vi "FindAndTrackFaces.vi"(7 "Check face":bool, 8 "error in (no error)":errorcluster, 10 "Image in":T1, 11 "Object Tracking Session In":T2) -> (0 "error out":errorcluster, 1 "Face Images":T1[](array[typedef]), 2 "Image out":T1(plugin-control), 3 "Object Tracking Session Out":T2)   [LabVIEW 2019]
uses:
  <vilib>/vision/Image Controls.llb/IMAQ Image.ctl
  <vilib>/vision/Tracking.llb/IMAQ Object Tracking Session.ctl
panel:
  out "size(s)":i32
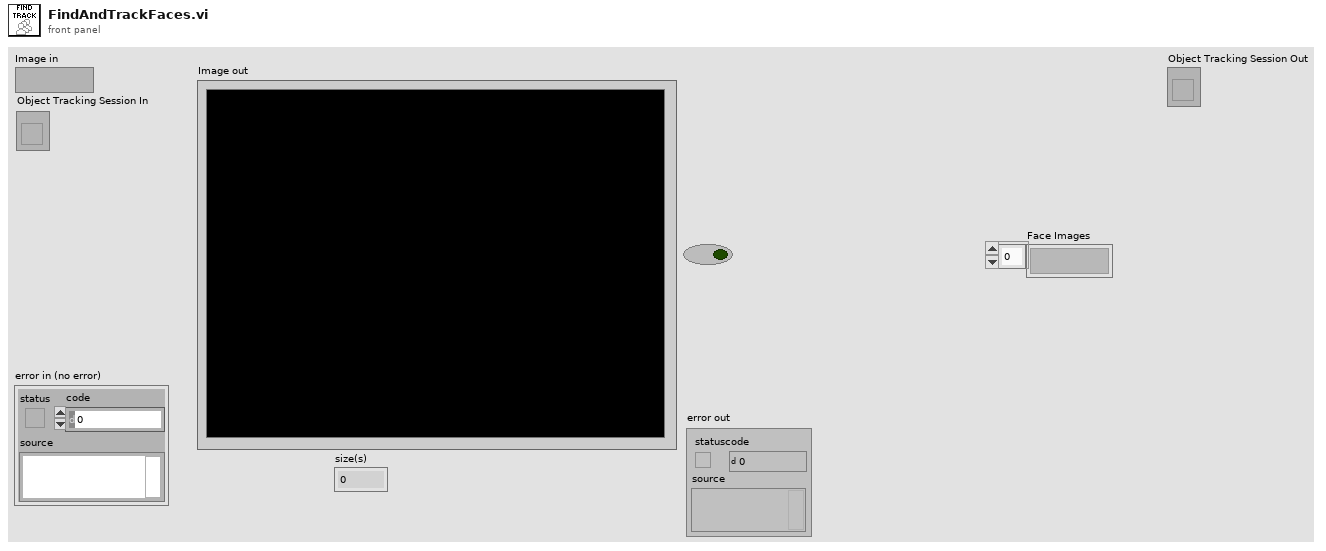
[diagram p1: front panel]
types:
  T1 = typedef "IMAQ Image.ctl" = refnum<image>
  T2 = typedef "IMAQ Object Tracking Session.ctl" = refnum<k20>
  T3 = typedef "IMAQ Rectangle" = cluster{"Left":i32, "Top":i32, "Right":i32, "Bottom":i32, "Rotation":dbl}
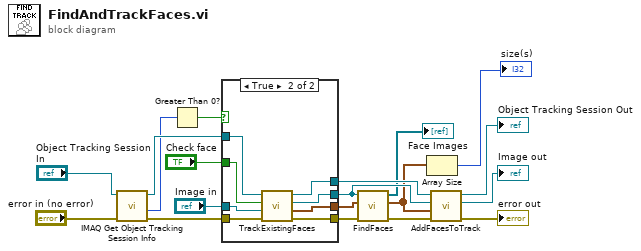
[diagram p0: block diagram]
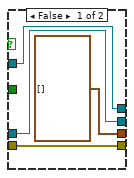
[diagram p2: hidden frame]
diagram:
  n1 = call "IMAQ Get Object Tracking Session Info"("error in (no error)"="error in (no error)", "Object Tracking Session In"="Object Tracking Session In") -> ("error out"=w10:errorcluster, "Number of Objects"=w11:i32, "Object Tracking Session Out"=w13:T2)  [unwired: 6 in, 1 out]
  n2 = Greater Than 0?(x=w11) -> (x > 0?=w12:bool)
  n3 = case shown="True" w12 {
    tunnel: "Image in" -> [w22 w31]
    tunnel: w13 -> [w23 w30]
    tunnel: w10 -> [w21 w29]
    tunnel: [w21 w28] -> w18
    tunnel: [w22 w27] -> w9
    tunnel: [w23 w26] -> w16
    tunnel: [T3[] [] w25] -> w8
    tunnel: "Check face" -> [_ w24]
    frame False {
    }
    frame True {
      n4 = call "TrackExistingFaces.vi"("error in (no error)"=w29, "Image in"=w31, "Check face"=w24, "Refnum in"=w30) -> ("error out"=w28:errorcluster, "Array"=w25:T3[], "Image (duplicate)"=w27:T1, "Refnum out"=w26:T2)  [unwired: 4 in]
    }
  }
  n5 = call "FindFaces.vi"("error in"=w18, "Faces In"=w8, "Image In"=w9) -> ("error out"=w15:errorcluster, "Faces"=w1:T3[], "Array"=→"Face Images":T1[])  [unwired: 6 in]
  n6 = Array Size(array=w1) -> (size(s)=→"size(s)":i32)
  n7 = call "AddFacesToTrack.vi"("error in (no error)"=w15, "Faces"=w1, "Image (duplicate) in"=w9, "Refnum in"=w16) -> ("error out"=→"error out":errorcluster, "Image (duplicate) out"=→"Image out":T1, "Refnum out"=→"Object Tracking Session Out":T2)  [unwired: 5 in]
